vi "Get Default Type Formatting.vi"() -> (0 "Default Type Formatting":T1)   [LabVIEW 2011]
uses:
  Options API/Private/EasyXML Options - Type Formatting Cluster.ctl
  Type Defs/Formatting Data Type -- Enum.ctl
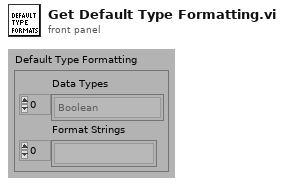
[diagram p1: front panel]
types:
  T1 = typedef "EasyXML Options - Type Formatting Cluster.ctl" = cluster{"Data Types":T2[], "Format Strings":string[]}
  T2 = typedef "Formatting Data Type -- Enum.ctl" = enum16{"<unknown>", "Cluster", "Array", "String", "Path", "Boolean", "Time Stamp", "Enum", "Numeric - EXT", "Numeric - DBL", "Numeric - SGL", "Numeric - I64", "Numeric - I32", "Numeric - I16", "Numeric - I8", "Numeric - U64", "Numeric - U32", "Numeric - U16", "Numeric - U8", "Numeric - CXT", "Numeric - CDB", "Numeric - CSG", "VISA Resource"}
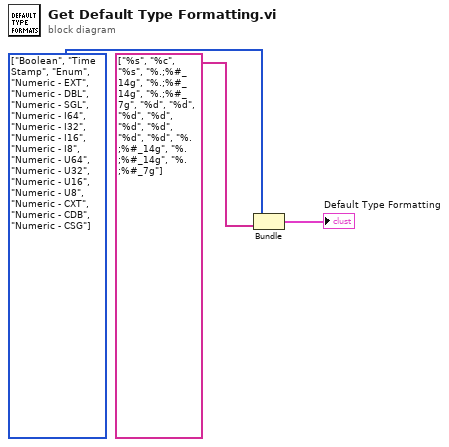
[diagram p0: block diagram]
diagram:
  w2 = T2[] [enum."Boolean", enum."Time Stamp", enum."Enum", enum."Numeric - EXT", enum."Numeric - DBL", enum."Numeric - SGL", enum."Numeric - I64", enum."Numeric - I32", enum."Numeric - I16", enum."Numeric - I8", enum."Numeric - U64", enum."Numeric - U32", enum."Numeric - U16", enum."Numeric - U8", enum."Numeric - CXT", enum."Numeric - CDB", enum."Numeric - CSG"] items=["<unknown>", "Cluster", "Array", "String", "Path", "Boolean", "Time Stamp", "Enum", "Numeric - EXT", "Numeric - DBL", "Numeric - SGL", "Numeric - I64", "Numeric - I32", "Numeric - I16", "Numeric - I8", "Numeric - U64", "Numeric - U32", "Numeric - U16", "Numeric - U8", "Numeric - CXT", "Numeric - CDB", "Numeric - CSG", "VISA Resource"]
  n1 = Bundle(w2, "Item Names"=string[] ["%s", "%c", "%s", "%.;%#_14g", "%.;%#_14g", "%.;%#_7g", "%d", "%d", "%d", "%d", "%d", "%d", "%d", "%d", "%.;%#_14g", "%.;%#_14g", "%.;%#_7g"]) -> (→"Default Type Formatting":cluster{T2[], "Item Names":string[]})  [unwired: 1 in]
